vi "Integration.vi"() -> ()   [LabVIEW 2020]
uses:
  <vilib>/express/express arith-compare/Formula/XNode/ExpressFormulaBlockNode.xnode
panel:
  out "Offset vol 2":dbl
  out "Z_in":dbl
  out "Z_vol":dynamicdata(graph)
  out "X_in":dbl
  out "X_vol":dynamicdata(graph)
  in  "Gain(Acc)":dbl
  in  "Gain(Gyro)":dbl
  out "PITCH(comp)":dbl(knob) scale=-90.0..90.0
  out "PITCH after":dbl(graph)
  out "YAW각":dbl
  out "PITCH각":dbl
  out "PITCH(gyro)":dbl(knob) scale=-90.0..90.0
  out "X_offset":dbl
  out "Z_offset":dbl
  out "dt":dbl
  out "t2":dbl
  out "t1":dbl
  in  "정지":bool
  in  "Offset(Gyro)":bool
  out "YAW":dbl(knob) scale=-90.0..90.0
  out "순간 YAW":dbl
  out "순간 PITCH":dbl
  in  "감도(자이로)":dbl
  out "?":dbl(graph)
  in  "Sensitivity(가속도)":dbl
  out "180/pi":dbl
  out "Pitch(acc)":dbl(knob) scale=-90.0..90.0
  out "Z-vol":dbl
  out "?":dynamicdata(graph)
  out "X-vol":dbl
  out "?":dynamicdata(graph)
  out "Offset vol":dbl
  in  "Offset(Acc)":bool
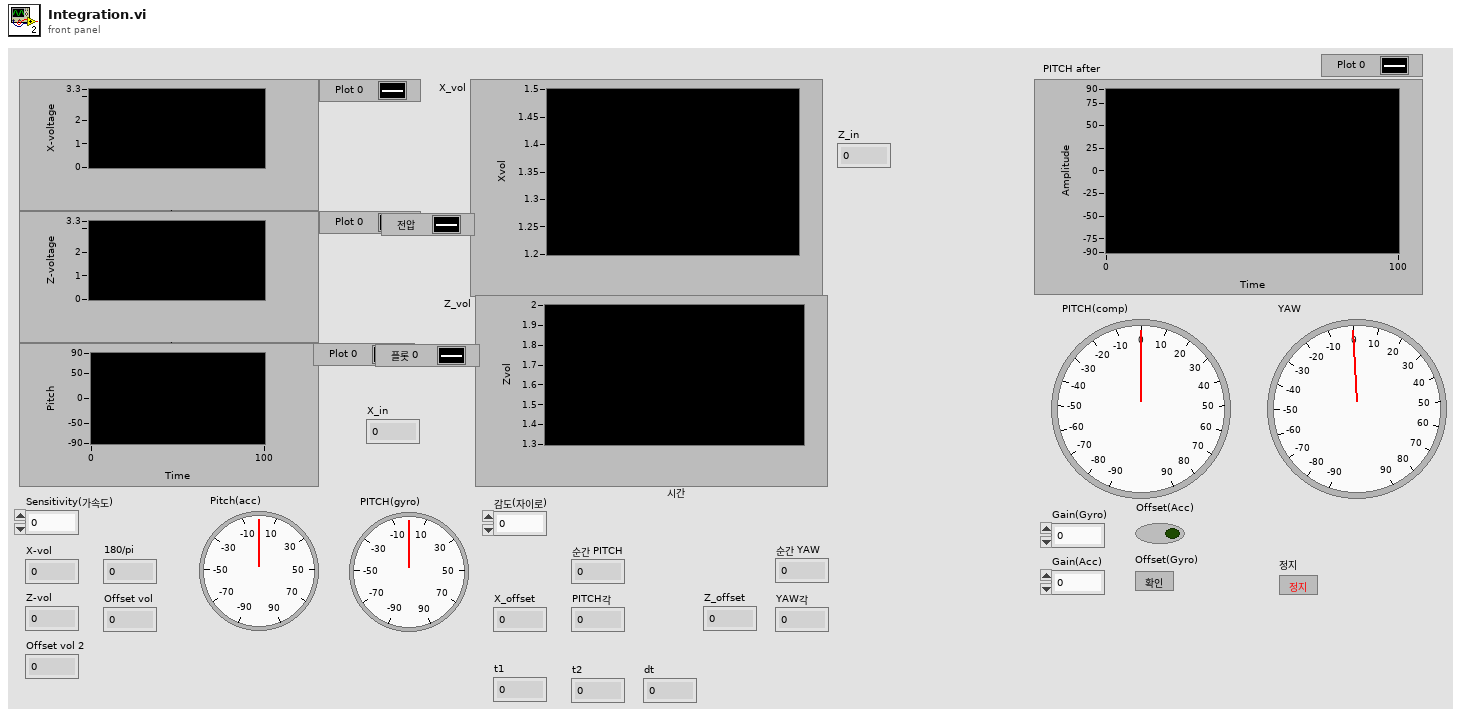
[diagram p1: front panel]
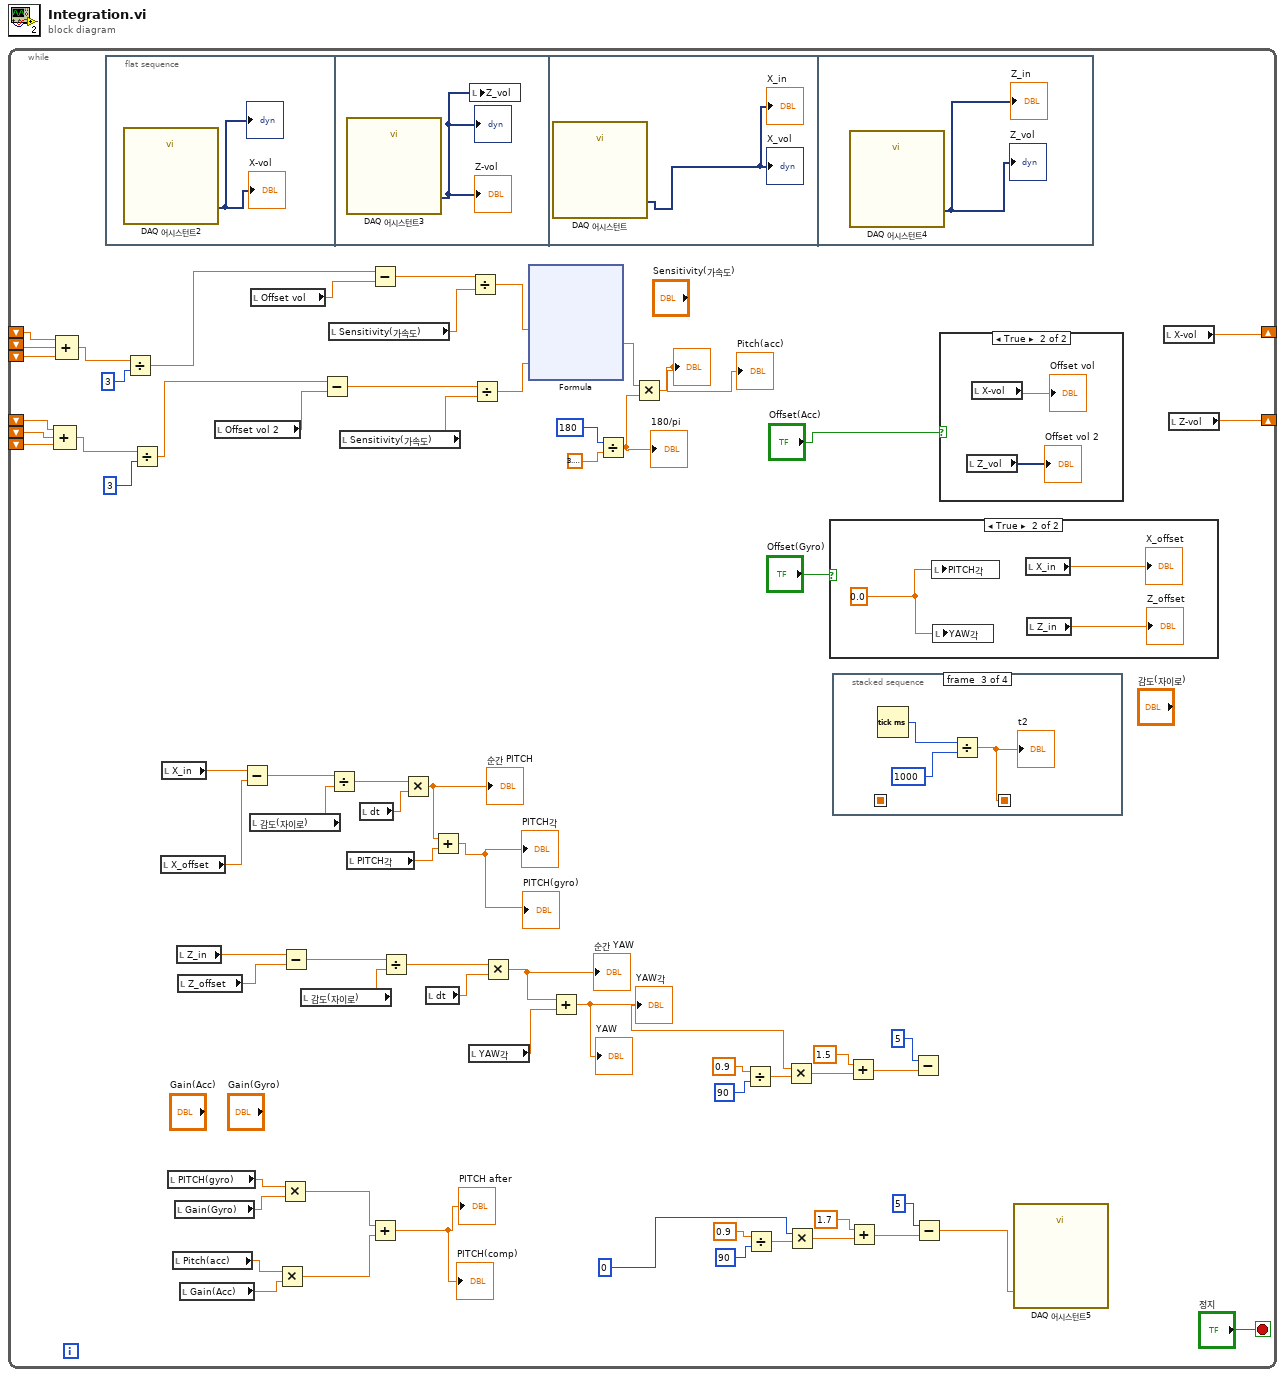
[diagram p0: block diagram]
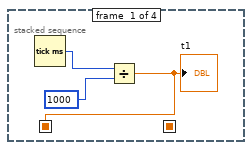
[diagram p3: hidden frame]
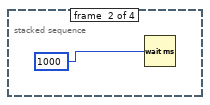
[diagram p4: hidden frame]
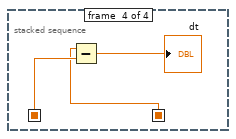
[diagram p5: hidden frame]
diagram:
  n1 = while {
    shift-right: [w17] -> _
    shift-left: _ -> [w15]
    shift-right: [w16] -> _
    shift-left: _ -> [w12]
    shift-left: _ -> [w14]
    shift-left: _ -> [w13]
    shift-left: _ -> [w11]
    shift-left: _ -> [w10]
    stop <- "정지" stop-if-true
    n2 = Compound Arithmetic op=ADD(w12, w11, w10) -> (w8:dbl)
    n3 = Compound Arithmetic op=ADD(w15, w14, w13) -> (w9:dbl)
    n4 = flat-sequence {
      frame #0 {
        n5 = call "DAQ 어시스턴트2"() -> ("data"=→"X-vol" →"?":dynamicdata)  [unwired: 17 in, 2 out]
      }
      frame #1 {
        n6 = call "DAQ 어시스턴트3"() -> ("data"=w98:dynamicdata)  [unwired: 17 in, 2 out]
        "Z-vol" <- w98
        "?" <- w98
        n7 = local write "Z_vol"(w98) -> ()
      }
      frame #2 {
        n8 = call "DAQ 어시스턴트"() -> ("data"=→"X_vol" →"X_in":dynamicdata)  [unwired: 17 in, 2 out]
      }
      frame #3 {
        n9 = call "DAQ 어시스턴트4"() -> ("data"=→"Z_vol" →"Z_in":dynamicdata)  [unwired: 17 in, 2 out]
      }
    }
    n10 = Divide(x=w9, y=3) -> (x/y=w5:dbl)
    n11 = Divide(x=w8, y=3) -> (x/y=w4:dbl)
    n12 = local read "X_offset"() -> (w58:dbl)
    n13 = local read "X_in"() -> (w41:dbl)
    n14 = local read "PITCH(gyro)"() -> (w39:dbl)
    n15 = local read "Pitch(acc)"() -> (w37:dbl)
    n16 = local read "Gain(Gyro)"() -> (w38:dbl)
    n17 = local read "Z_in"() -> (w40:dbl)
    n18 = local read "Z_offset"() -> (w53:dbl)
    n19 = local read "Gain(Acc)"() -> (w36:dbl)
    n20 = local read "Offset vol 2"() -> (w68:dbl)
    n21 = Subtract(x=w41, y=w58) -> (x-y=w57:dbl)
    n22 = local read "감도(자이로)"() -> (w56:dbl)
    n23 = local read "Offset vol"() -> (w71:dbl)
    n24 = Multiply(x=w37, y=w36) -> (x*y=w34:dbl)
    n25 = Multiply(x=w39, y=w38) -> (x*y=w35:dbl)
    n26 = Subtract(x=w40, y=w53) -> (x-y=w52:dbl)
    n27 = local read "감도(자이로)"() -> (w51:dbl)
    n28 = Subtract(x=w4, y=w68) -> (x-y=w66:dbl)
    n29 = local read "Sensitivity(가속도)"() -> (w69:dbl)
    n30 = Divide(x=w57, y=w56) -> (x/y=w48:dbl)
    n31 = local read "Sensitivity(가속도)"() -> (w67:dbl)
    n32 = local read "PITCH각"() -> (w54:dbl)
    n33 = local read "dt"() -> (w55:dbl)
    n34 = Subtract(x=w5, y=w71) -> (x-y=w70:dbl)
    n35 = Add(x=w35, y=w34) -> (x+y=→"PITCH after" →"PITCH(comp)":dbl)
    n36 = Divide(x=w52, y=w51) -> (x/y=w47:dbl)
    n37 = Multiply(x=w48, y=w55) -> (x*y=w44:dbl)
    "순간 PITCH" <- w44
    n38 = local read "dt"() -> (w50:dbl)
    n39 = Add(x=w44, y=w54) -> (x+y=→"PITCH(gyro)" →"PITCH각":dbl)
    n40 = local read "YAW각"() -> (w49:dbl)
    n41 = Divide(x=w70, y=w69) -> (x/y=w61:dbl)
    n42 = Divide(x=w66, y=w67) -> (x/y=w60:dbl)
    n43 = Multiply(x=w47, y=w50) -> (x*y=w45:dbl)
    "순간 YAW" <- w45
    n44 = xnode "Formula"("X_vol"=w61, "Z_vol"=w60) -> ("결과"=w63:dbl)  [unwired: 1 in, 1 out]
    n45 = Add(x=w45, y=w49) -> (x+y=w19:dbl)
    "YAW" <- w19
    "YAW각" <- w19
    n46 = Divide(x=180, y=3.141592653589793) -> (x/y=w62:dbl)
    "180/pi" <- w62
    n47 = Multiply(x=w63, y=w62) -> (x*y=→"?" →"Pitch(acc)":dbl)
    n48 = Divide(x=0.9, y=90) -> (x/y=w24:dbl)
    n49 = Divide(x=0.9, y=90) -> (x/y=w31:dbl)
    n50 = Multiply(x=w19, y=w24) -> (x*y=w23:dbl)
    n51 = Multiply(x=0, y=w31) -> (x*y=w30:dbl)
    n52 = case shown="True" "Offset(Gyro)" {
      frame False {
      }
      frame True {
        w72 = 0.0
        n53 = local write "PITCH각"(w72) -> ()
        n54 = local write "YAW각"(w72) -> ()
        n55 = local read "X_in"() -> (→"X_offset":dbl)
        n56 = local read "Z_in"() -> (→"Z_offset":dbl)
      }
    }
    n57 = stacked-sequence {
      seq-local: [w75 _ _ _] -> [_ _ _ w83]
      seq-local: [_ _ w79 _] -> [_ _ _ w82]
      frame #0 {
        n58 = Tick Count (ms)() -> (millisecond timer value=w77:u32)
        n59 = Divide(x=w77, y=1000) -> (x/y=w75:dbl)
        "t1" <- w75
      }
      frame #1 {
        n60 = Wait (ms)(milliseconds to wait=1000) -> ()  [unwired: 1 out]
      }
      frame #2 {
        n61 = Tick Count (ms)() -> (millisecond timer value=w81:u32)
        n62 = Divide(x=w81, y=1000) -> (x/y=w79:dbl)
        "t2" <- w79
      }
      frame #3 {
        n63 = Subtract(x=w82, y=w83) -> (x-y=→"dt":dbl)
      }
    }
    n64 = Add(x=1.5, y=w23) -> (x+y=w20:dbl)
    n65 = Add(x=1.7, y=w30) -> (x+y=w27:dbl)
    n66 = Subtract(x=5, y=w20) -> ()  [unwired: 1 out]
    n67 = Subtract(x=5, y=w27) -> (x-y=w2:dbl)
    n68 = case shown="True" "Offset(Acc)" {
      frame False {
      }
      frame True {
        n69 = local read "Z_vol"() -> (→"Offset vol 2":dynamicdata)
        n70 = local read "X-vol"() -> (→"Offset vol":dbl)
      }
    }
    n71 = call "DAQ 어시스턴트5"("data"=w2) -> ()  [unwired: 17 in, 2 out]
    n72 = local read "X-vol"() -> (w17:dbl)
    n73 = local read "Z-vol"() -> (w16:dbl)
  }
